vi "Make Measurements Visible.vi"(7 "Item":T1, 8 "error in (no error)":errorcluster, 10 "Visible?":bool=TRUE, 11 "Measurements Ref":refnum<vi>) -> (0 "error out":errorcluster)   [LabVIEW 2018]
uses:
  Controls/Measurement Selector.ctl
  Controls/Measurements.ctl
  Controls/Channel Measurement String Control.ctl
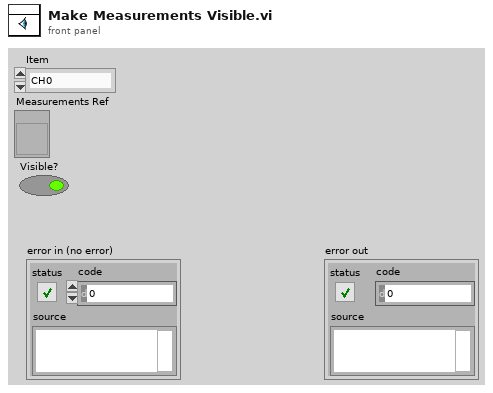
[diagram p1: front panel]
types:
  T1 = typedef "Measurement Selector.ctl" = enum16{"CH0", "CH1", "Cursors"}
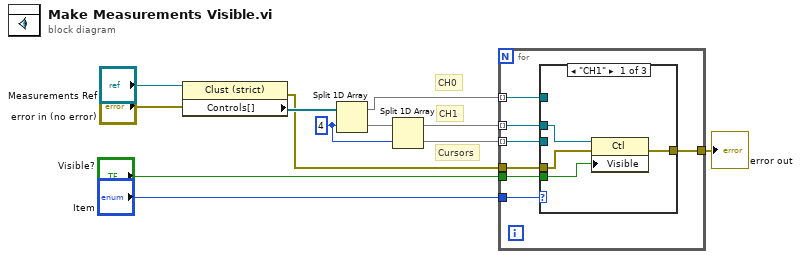
[diagram p0: block diagram]
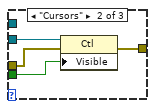
[diagram p2: hidden frame]
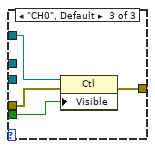
[diagram p3: hidden frame]
diagram:
  w10 = 4 ("index")
  # "CH0"
  # "Cursors"
  # "CH1"
  n1 = property class="Clust (strict)"(reference="Measurements Ref", error in="error in (no error)") -> (error out=w2:errorcluster, "Controls[]"=w12:refnum<vi>[])  [unwired: 1 out]
  n2 = Split 1D Array(array=w12, index=w10) -> (first subarray=w7:refnum<vi>[], second subarray=w11:refnum<vi>[])
  n3 = Split 1D Array(array=w11, index=w10) -> (first subarray=w9:refnum<vi>[], second subarray=w8:refnum<vi>[])
  n4 = for {
    tunnel: w9 -> [w18] mode=indexing
    tunnel: w8 -> [w17] mode=indexing
    tunnel: w7 -> [w19] mode=indexing
    tunnel: "Item" -> [w16]
    tunnel: "Visible?" -> [w15]
    tunnel: w2 -> [w14]
    tunnel: [w13] -> w1
    n5 = case shown="\"CH1\"" w16 {
      tunnel: w19 -> [_ _ w30]
      tunnel: w18 -> [w22 _ _]
      tunnel: w17 -> [_ w26 _]
      tunnel: w15 -> [w23 w27 w31]
      tunnel: w14 -> [w20 w25 w29]
      tunnel: [w21 w24 w28] -> w13
      frame "CH1" {
        n6 = property class="Ctl"(reference=w22, error in=w20, "Visible"=w23) -> (error out=w21:errorcluster)  [unwired: 1 out]
      }
      frame "Cursors" {
        n7 = property class="Ctl"(reference=w26, error in=w25, "Visible"=w27) -> (error out=w24:errorcluster)  [unwired: 1 out]
      }
      frame "CH0", Default {
        n8 = property class="Ctl"(reference=w30, error in=w29, "Visible"=w31) -> (error out=w28:errorcluster)  [unwired: 1 out]
      }
    }
  }
  "error out" <- w1
